vi "Delete Folder via Commandline.vi"(8 "error in (no error)":errorcluster, 11 "Path":path) -> (0 "error out":errorcluster, 3 "Path out":path)   [LabVIEW 2016, in "SLL File IO.lvlib"]
doc: "Opens a File or Folder or EXE depending on the path specified."
uses:
  SLL File IO.lvlib
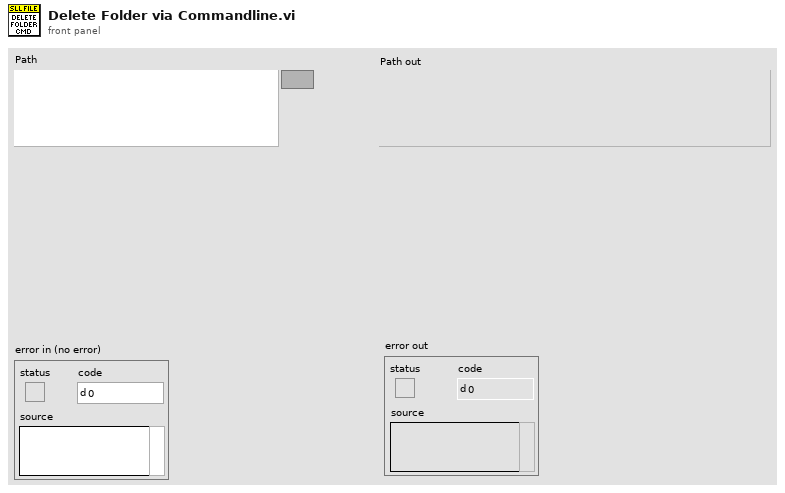
[diagram p1: front panel]
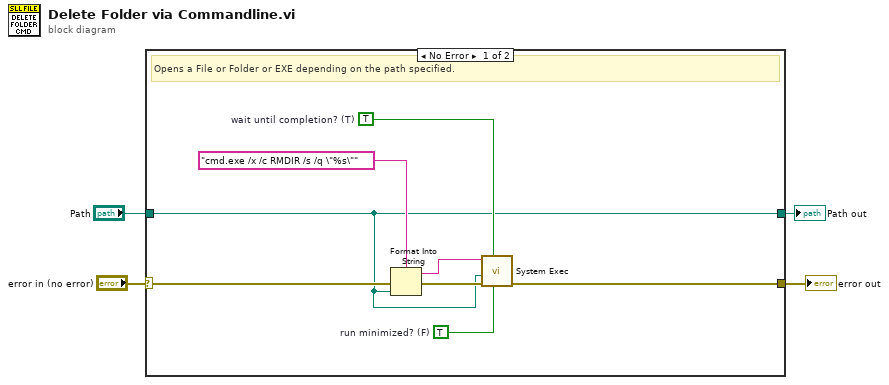
[diagram p0: block diagram]
diagram:
  n1 = case shown="No Error" "error in (no error)" {
    selector: "error in (no error)" -> [w12 w13]
    tunnel: [w11 w13] -> w3
    tunnel: "Path" -> [w5 _]
    tunnel: [w5 _] -> w1
    frame No Error {
      w9 = TRUE  # run minimized? (F)
      w10 = TRUE  # wait until completion? (T)
      # "Opens a File or Folder or EXE depending on the path specified."
      n2 = Format Into String(format string="cmd.exe /x /c RMDIR /s /q \"%s\"", error in=w12, w5) -> (resulting string=w6:string, error out=w8:errorcluster)  [unwired: 1 in]
      n3 = call <vilib>:"System Exec.vi"("run minimized? (F)"=w9, "wait until completion? (T)"=w10, "error in (no error)"=w8, "working directory"=w5, "command line"=w6) -> ("error out"=w11:errorcluster)  [unwired: 3 in, 3 out]
    }
    frame Error {
    }
  }
  "error out" <- w3
  "Path out" <- w1
